vi "VI controls.vi"(8 "error in (no error)":errorcluster, 11 "VI refnums":refnum<vi>[](array[refnum])) -> (0 "error out":errorcluster, 2 "all Label text":string[](array[string]), 3 "VI controls":refnum<vi>[](array[refnum]))   [LabVIEW 2015]
panel:
  out "sorted array":cluster{"Label.Text":string, i32}[](array[cluster])
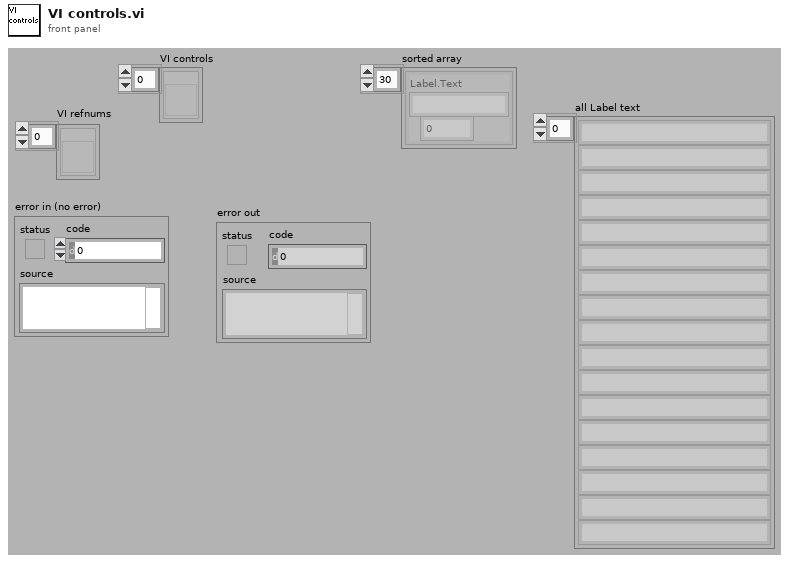
[diagram p1: front panel]
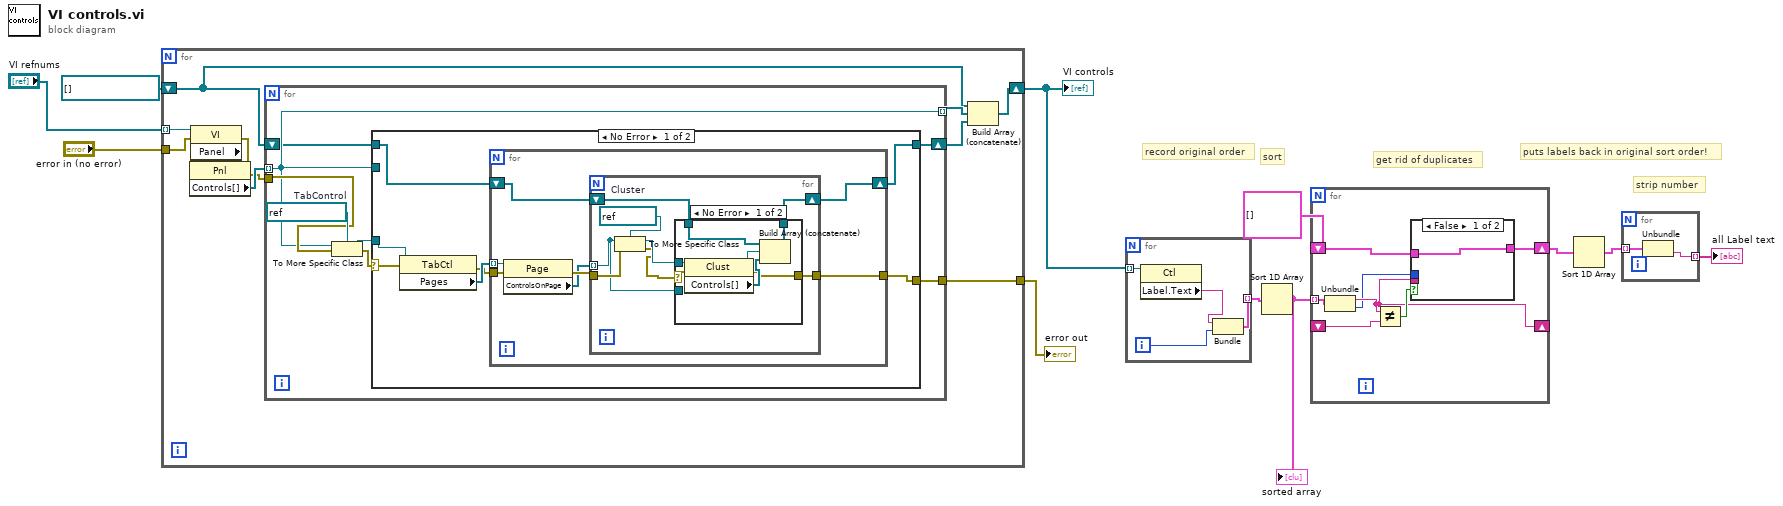
[diagram p0: block diagram]
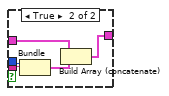
[diagram p2: hidden frame]
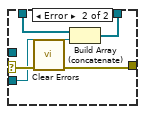
[diagram p3: hidden frame]
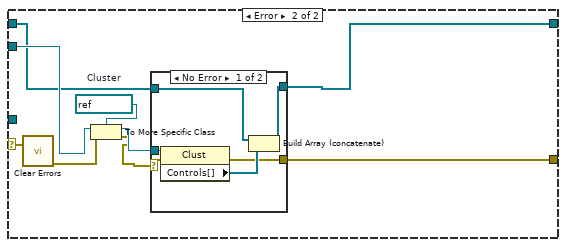
[diagram p4: hidden frame]
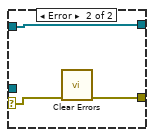
[diagram p5: hidden frame]
diagram:
  # "strip number"
  # "record original order"
  # "puts labels back in original sort order!"
  # "sort"
  # "get rid of duplicates"
  n1 = for {
    shift-right: [w18] -> w11
    shift-left: refnum<vi>[] [] -> [w14]
    tunnel: "VI refnums" -> [w17] mode=indexing
    tunnel: "error in (no error)" -> [w16]
    tunnel: [w12] -> w8
    n2 = property class="VI"(reference=w17, error in=w16) -> (error out=w19:errorcluster, "Panel"=w22:refnum<vi>)  [unwired: 1 out]
    n3 = property class="Pnl"(reference=w22, error in=w19) -> (error out=w20:errorcluster, "Controls[]"=w21:refnum<vi>[])  [unwired: 1 out]
    n4 = for {
      tunnel: w21 -> [w26] mode=indexing
      tunnel: w20 -> [w27]
      shift-right: [w24] -> w13
      shift-left: w14 -> [w25]
      tunnel: [w26] -> w15 mode=indexing
      tunnel: [w23] -> w12
      w30 = refnum<vi> refnum  # TabControl
      n5 = To More Specific Class(target class=w30, reference=w26, error in=w27) -> (specific class reference=w29:refnum<vi>, error out=w28:errorcluster)
      n6 = case shown="No Error" w28 {
        selector: w28 -> [w36 w72]
        tunnel: w29 -> [w37 _]
        tunnel: w26 -> [_ w73]
        tunnel: w25 -> [w33 w70]
        tunnel: [w32 w69] -> w24
        tunnel: [w31 w65] -> w23
        frame No Error {
          n7 = property class="TabCtl"(reference=w37, error in=w36) -> (error out=w34:errorcluster, "Pages"=w35:refnum<vi>[])  [unwired: 1 out]
          n8 = for {
            tunnel: w34 -> [w44]
            tunnel: w35 -> [w43] mode=indexing
            shift-right: [w38] -> w32
            shift-left: w33 -> [w41]
            tunnel: [w39] -> w31
            n9 = property class="Page"(reference=w43, error in=w44) -> (error out=w42:errorcluster, "ControlsOnPage"=w40:refnum<vi>[])  [unwired: 1 out]
            n10 = for {
              tunnel: w40 -> [w45] mode=indexing
              tunnel: w42 -> [w50]
              shift-right: [w47] -> w38
              shift-left: w41 -> [w48]
              tunnel: [w46] -> w39
              w52 = refnum<vi> refnum  # Cluster
              n11 = To More Specific Class(target class=w52, reference=w45, error in=w50) -> (specific class reference=w51:refnum<vi>, error out=w49:errorcluster)
              n12 = case shown="No Error" w49 {
                selector: w49 -> [w58 w63]
                tunnel: w51 -> [w59 _]
                tunnel: w48 -> [w54 w64]
                tunnel: [w56 w61] -> w47
                tunnel: [w55 w62] -> w46
                tunnel: w45 -> [_ w60]
                frame No Error {
                  n13 = property class="Clust"(reference=w59, error in=w58) -> (reference out=w53:refnum<vi>, error out=w55:errorcluster, "Controls[]"=w57:refnum<vi>[])
                  n14 = Build Array (concatenate)(w54, w53, w57) -> (w56:refnum<vi>[])
                }
                frame Error {
                  n15 = call <vilib>:"Clear Errors.vi"("error in (no error)"=w63) -> ("error out"=w62:errorcluster)  [unwired: 5 in, 1 out]
                  n16 = Build Array (concatenate)(w64, w60) -> (w61:refnum<vi>[])
                }
              }
            }
          }
        }
        frame Error {
          w68 = refnum<vi> refnum  # Cluster
          n17 = call <vilib>:"Clear Errors.vi"("error in (no error)"=w72) -> ("error out"=w71:errorcluster)  [unwired: 5 in, 1 out]
          n18 = To More Specific Class(target class=w68, reference=w73, error in=w71) -> (specific class reference=w67:refnum<vi>, error out=w66:errorcluster)
          n19 = case shown="No Error" w66 {
            selector: w66 -> [w78 w81]
            tunnel: w67 -> [w79 _]
            tunnel: w70 -> [w76 w82]
            tunnel: [w75 w82] -> w69
            tunnel: [w74 w80] -> w65
            frame No Error {
              n20 = property class="Clust"(reference=w79, error in=w78) -> (error out=w74:errorcluster, "Controls[]"=w77:refnum<vi>[])  [unwired: 1 out]
              n21 = Build Array (concatenate)(w76, w77) -> (w75:refnum<vi>[])
            }
            frame Error {
              n22 = call <vilib>:"Clear Errors.vi"("error in (no error)"=w81) -> ("error out"=w80:errorcluster)  [unwired: 5 in, 1 out]
            }
          }
        }
      }
    }
    n23 = Build Array (concatenate)(w14, w15, w13) -> (w18:refnum<vi>[])
  }
  "VI controls" <- w11
  "error out" <- w8
  n24 = for {
    tunnel: w11 -> [w86] mode=indexing
    tunnel: [w84] -> w6 mode=indexing
    i -> [w85]
    n25 = property class="Ctl"(reference=w86) -> ("Label.Text"=w83:string)  [unwired: 1 in, 2 out]
    n26 = Bundle("Label.Text"=w83, w85) -> (w84:cluster{"Label.Text":string, i32})  [unwired: 1 in]
  }
  n27 = Sort 1D Array(array=w6) -> (sorted array=w5:cluster{"Label.Text":string, i32}[])
  "sorted array" <- w5
  n28 = for {
    tunnel: w5 -> [w89] mode=indexing
    shift-right: [w88] -> _
    shift-left: _ -> [w93]
    shift-right: [w90] -> w4
    shift-left: cluster{i32, "Label.Text":string}[] [] -> [w91]
    n29 = Unbundle(w89) -> ("Label.Text"=w88:string, w87:i32)
    n30 = Not Equal?(x=w88, y=w93) -> (x != y?=w92:bool)
    n31 = case shown="False" w92 {
      tunnel: w91 -> [w94 w99]
      tunnel: [w94 w98] -> w90
      tunnel: w88 -> [_ w97]
      tunnel: w87 -> [_ w95]
      frame False {
      }
      frame True {
        n32 = Bundle(w95, "Label.Text"=w97) -> (w96:cluster{i32, "Label.Text":string})  [unwired: 1 in]
        n33 = Build Array (concatenate)(w99, w96) -> (w98:cluster{i32, "Label.Text":string}[])
      }
    }
  }
  n34 = Sort 1D Array(array=w4) -> (sorted array=w3:cluster{i32, "Label.Text":string}[])
  n35 = for {
    tunnel: w3 -> [w101] mode=indexing
    tunnel: [w100] -> w2 mode=indexing
    n36 = Unbundle(w101) -> ("Label.Text"=w100:string)  [unwired: 1 out]
  }
  "all Label text" <- w2
